vi "RTS Read Custom Commands.vi"(8 "Error In":errorcluster, 10 "Data Out":T1) -> (0 "Error Out":errorcluster, 2 "Custom Commands":string[](array[string]))   [LabVIEW 2016]
uses:
  Type Definitions/RTS TCP Multiple Connections Data.ctl
  Type Definitions/RTS TCP Commands.ctl
  <vilib>/Utility/error.llb/whitespace.ctl
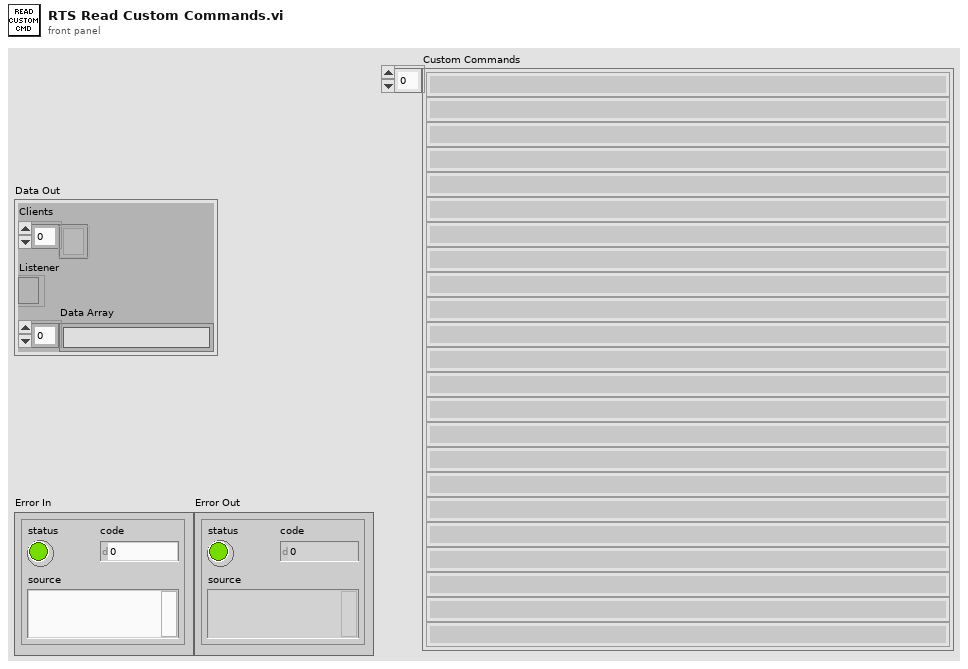
[diagram p1: front panel]
types:
  T1 = typedef "RTS TCP Multiple Connections Data.ctl" = cluster{"Clients":refnum<k5>[], "Listener":refnum<k5>, "Data Array":string[]}
  T2 = typedef "RTS TCP Commands.ctl" = string
  T3 = typedef "whitespace.ctl" = u16
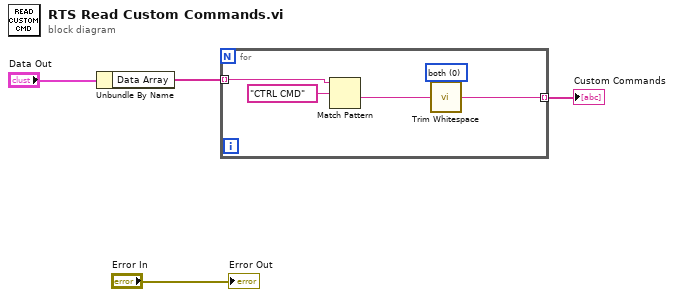
[diagram p0: block diagram]
diagram:
  n1 = Unbundle By Name("Data Out") -> ("Data Array"=w2:string[])
  n2 = for {
    tunnel: w2 -> [w9] mode=indexing
    tunnel: [w6] -> w1 mode=indexing
    w5 = T3 0 items=["both", "start of string", "end of string"] ("location (both)")
    n3 = Match Pattern(string=w9, regular expression=T2 "CTRL CMD" ("TCP Commands")) -> (after substring=w7:string)  [unwired: 1 in, 3 out]
    n4 = call <vilib>:"Trim Whitespace.vi"("string"=w7, "location (both)"=w5) -> ("trimmed string"=w6:string)
  }
  "Custom Commands" <- w1
  "Error Out" <- "Error In"
